vi "Guitar Subvi.vi"(0 "error out":errorcluster, 1 "Image Dst Out":T1, 2 "Blue Guitar 2":T2={"Global Rectangle"=[569, 290, 594, 372], "Contours"=[{"ID"=enum."External", "Type"=2, "Coordinates"=[593, 371, 569, 290]}]} {"Contours"."Type" items=["No Selection", "Point", "Line", "Rectangle", "Oval", "Polygon", "Freehand Region", "Annulus", "Unused2", "Unused3", "Broken Line", "Freehand Line", "Rotated Rectangle"]}, 3 "Yellow Guitar 2":T2={"Global Rectangle"=[546, 282, 563, 376], "Contours"=[{"ID"=enum."External", "Type"=2, "Coordinates"=[562, 375, 546, 282]}]} {"Contours"."Type" items=["No Selection", "Point", "Line", "Rectangle", "Oval", "Polygon", "Freehand Region", "Annulus", "Unused2", "Unused3", "Broken Line", "Freehand Line", "Rotated Rectangle"]}, 4 "Green Guitar 2":T2={"Global Rectangle"=[498, 284, 505, 376], "Contours"=[{"ID"=enum."External", "Type"=2, "Coordinates"=[498, 375, 504, 284]}]} {"Contours"."Type" items=["No Selection", "Point", "Line", "Rectangle", "Oval", "Polygon", "Freehand Region", "Annulus", "Unused2", "Unused3", "Broken Line", "Freehand Line", "Rotated Rectangle"]}, 5 "Red Guitar 2":T2={"Global Rectangle"=[526, 284, 530, 370], "Contours"=[{"ID"=enum."External", "Type"=2, "Coordinates"=[529, 369, 526, 284]}]} {"Contours"."Type" items=["No Selection", "Point", "Line", "Rectangle", "Oval", "Polygon", "Freehand Region", "Annulus", "Unused2", "Unused3", "Broken Line", "Freehand Line", "Rotated Rectangle"]}, 6 "Orange Guitar 2":T2={"Global Rectangle"=[587, 282, 628, 378], "Contours"=[{"ID"=enum."External", "Type"=2, "Coordinates"=[627, 377, 587, 282]}]} {"Contours"."Type" items=["No Selection", "Point", "Line", "Rectangle", "Oval", "Polygon", "Freehand Region", "Annulus", "Unused2", "Unused3", "Broken Line", "Freehand Line", "Rotated Rectangle"]}) -> (11 "Orange Guitar LED":bool, 13 "Red Guitar LED":bool, 15 "Green Guitar LED":bool, 23 "Blue Guitar LED":bool, 24 "Yellow Guitar LED":bool)   [LabVIEW 2009]
uses:
  <vilib>/vision/Image Controls.llb/IMAQ Image.ctl
  <vilib>/Analysis/3filter.llb/Filter Passband Type.ctl
  <vilib>/Analysis/3filter.llb/Butterworth Filter (DBL).vi
  <vilib>/Analysis/NI_AALBase.lvlib
  <vilib>/vision/NI_Vision_Development_Module.lvlib
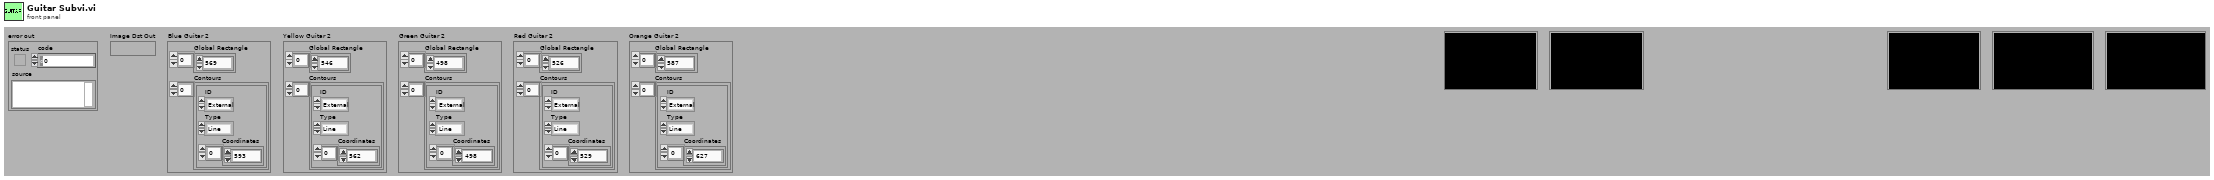
[diagram p1: front panel]
types:
  T1 = typedef "IMAQ Image.ctl" = refnum<image>
  T2 = cluster{"Global Rectangle":i32[], "Contours":cluster{"ID":enum32{"External", "Internal"}, "Type":u32, "Coordinates":i32[]}[]}
  T3 = typedef "NI_AALBase.lvlib/Filter Passband Type.ctl" = enum32{"Lowpass", "Highpass", "Bandpass", "Bandstop"}
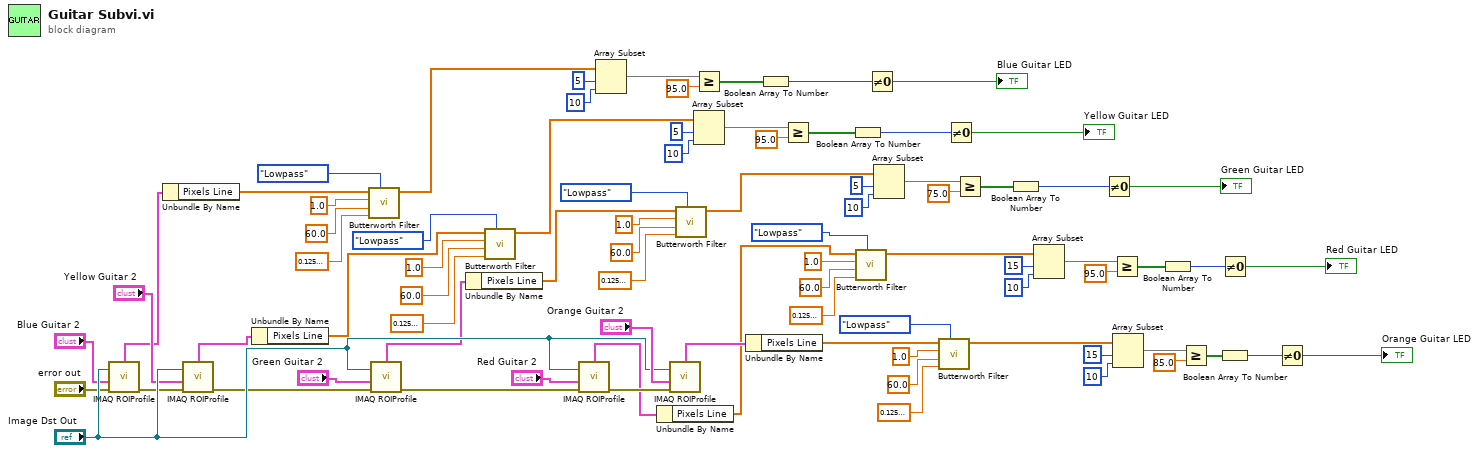
[diagram p0: block diagram]
diagram:
  n1 = call "IMAQ ROIProfile"("error in (no error)"="error out", "ROI Descriptor"="Blue Guitar 2", "Image"="Image Dst Out") -> ("error out"=w44:errorcluster, "ROI Graph"=w43:cluster{"x0":sgl, "dx":sgl, "Pixels Line":sgl[]})  [unwired: 4 out]
  n2 = Unbundle By Name(w43) -> ("Pixels Line"=w66:sgl[])
  n3 = call "IMAQ ROIProfile"("error in (no error)"=w44, "ROI Descriptor"="Yellow Guitar 2", "Image"="Image Dst Out") -> ("error out"=w14:errorcluster, "ROI Graph"=w47:cluster{"x0":sgl, "dx":sgl, "Pixels Line":sgl[]})  [unwired: 4 out]
  n4 = Unbundle By Name(w47) -> ("Pixels Line"=w50:sgl[])
  n5 = call-poly <vilib>:"Butterworth Filter.vi"("filter type"=Filter_Passband_Type."Lowpass", "low cutoff freq: fl"=0.12500000000000006 ("low 3"), "high cutoff freq: fh"=60.0 ("high 14"), "sampling freq: fs"=1.0 ("sampling  9"), "X"=w66) -> ("Filtered X"=w29:dbl[])  [unwired: 3 in, 1 out]
  n6 = call "IMAQ ROIProfile"("error in (no error)"=w14, "ROI Descriptor"="Green Guitar 2", "Image"="Image Dst Out") -> ("error out"=w15:errorcluster, "ROI Graph"=w41:cluster{"x0":sgl, "dx":sgl, "Pixels Line":sgl[]})  [unwired: 4 out]
  n7 = Unbundle By Name(w41) -> ("Pixels Line"=w38:sgl[])
  n8 = call-poly <vilib>:"Butterworth Filter.vi"("filter type"=Filter_Passband_Type."Lowpass", "low cutoff freq: fl"=0.12500000000000006 ("low  12"), "high cutoff freq: fh"=60.0 ("high 13"), "sampling freq: fs"=1.0 ("sampling 12"), "X"=w50) -> ("Filtered X"=w46:dbl[])  [unwired: 3 in, 1 out]
  n9 = call "IMAQ ROIProfile"("error in (no error)"=w15, "ROI Descriptor"="Red Guitar 2", "Image"="Image Dst Out") -> ("error out"=w74:errorcluster, "ROI Graph"=w17:cluster{"x0":sgl, "dx":sgl, "Pixels Line":sgl[]})  [unwired: 4 out]
  n10 = Array Subset(array=w29, index=5, length=10) -> (w60:dbl[])
  n11 = Unbundle By Name(w17) -> ("Pixels Line"=w20:sgl[])
  n12 = call "IMAQ ROIProfile"("error in (no error)"=w74, "ROI Descriptor"="Orange Guitar 2", "Image"="Image Dst Out") -> ("ROI Graph"=w75:cluster{"x0":sgl, "dx":sgl, "Pixels Line":sgl[]})  [unwired: 5 out]
  n13 = call-poly <vilib>:"Butterworth Filter.vi"("filter type"=Filter_Passband_Type."Lowpass", "low cutoff freq: fl"=0.12500000000000006 ("low  11"), "high cutoff freq: fh"=60.0 ("high 12"), "sampling freq: fs"=1.0 ("sampling 11"), "X"=w38) -> ("Filtered X"=w42:dbl[])  [unwired: 3 in, 1 out]
  n14 = Greater Or Equal?(x=w60, y=95.0) -> (x >= y?=w1:bool[])
  n15 = Array Subset(array=w46, index=5, length=10) -> (w55:dbl[])
  n16 = Unbundle By Name(w75) -> ("Pixels Line"=w10:sgl[])
  n17 = Boolean Array To Number(Boolean array=w1) -> (number=w58:u32)
  n18 = Greater Or Equal?(x=w55, y=95.0) -> (x >= y?=w53:bool[])
  n19 = Boolean Array To Number(Boolean array=w53) -> (number=w52:u32)
  n20 = call-poly <vilib>:"Butterworth Filter.vi"("filter type"=Filter_Passband_Type."Lowpass", "low cutoff freq: fl"=0.12500000000000006 ("low  10"), "high cutoff freq: fh"=60.0 ("high 11"), "sampling freq: fs"=1.0 ("sampling 10"), "X"=w20) -> ("Filtered X"=w16:dbl[])  [unwired: 3 in, 1 out]
  n21 = Not Equal To 0?(x=w58) -> (x != 0?=→"Blue Guitar LED":bool)
  n22 = Array Subset(array=w42, index=5, length=10) -> (w33:dbl[])
  n23 = call-poly <vilib>:"Butterworth Filter.vi"("filter type"=Filter_Passband_Type."Lowpass", "low cutoff freq: fl"=0.12500000000000006 ("low  9"), "high cutoff freq: fh"=60.0 ("high 10"), "sampling freq: fs"=1.0 ("sampling 9"), "X"=w10) -> ("Filtered X"=w13:dbl[])  [unwired: 3 in, 1 out]
  n24 = Not Equal To 0?(x=w52) -> (x != 0?=→"Yellow Guitar LED":bool)
  n25 = Greater Or Equal?(x=w33, y=75.0) -> (x >= y?=w35:bool[])
  n26 = Boolean Array To Number(Boolean array=w35) -> (number=w36:u32)
  n27 = Array Subset(array=w16, index=15, length=10) -> (w25:dbl[])
  n28 = Not Equal To 0?(x=w36) -> (x != 0?=→"Green Guitar LED":bool)
  n29 = Greater Or Equal?(x=w25, y=95.0) -> (x >= y?=w23:bool[])
  n30 = Array Subset(array=w13, index=15, length=10) -> (w5:dbl[])
  n31 = Boolean Array To Number(Boolean array=w23) -> (number=w22:u32)
  n32 = Greater Or Equal?(x=w5, y=85.0) -> (x >= y?=w7:bool[])
  n33 = Not Equal To 0?(x=w22) -> (x != 0?=→"Red Guitar LED":bool)
  n34 = Boolean Array To Number(Boolean array=w7) -> (number=w8:u32)
  n35 = Not Equal To 0?(x=w8) -> (x != 0?=→"Orange Guitar LED":bool)
